vi "Write condtional.vi"(5 "condtional":bool, 9 "ForLoop in":refnum<class "ForLoop.lvclass">) -> (3 "ForLoop out":refnum<class "ForLoop.lvclass">)   [LabVIEW 2014, in "ForLoop.lvclass"]
uses:
  ForLoop.lvclass
  ForLoop.lvclass/ForLoop.ctl
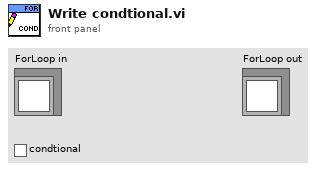
[diagram p1: front panel]
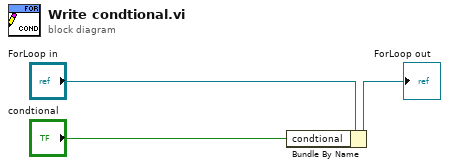
[diagram p0: block diagram]
diagram:
  n1 = Bundle By Name(cluster="ForLoop in", "condtional"="condtional") -> (→"ForLoop out":refnum<class "ForLoop.lvclass">)
